vi "None.vi"(8 "error in":errorcluster, 11 "ATM Data":T1={"UI Refs"={"Right Buttons"=refnum, "Left Buttons"=refnum, "User Input"=refnum, "ATM Messages"=refnum, "Left Menu"=refnum, "Right Menu"=refnum, "Enter"=refnum}, "Map"={}, "Login Valid?"=FALSE, "Queue Message"=refnum, "State"=enum."None", "User"={"Pin"="", "First Name"="", "Last Name"="", "Balance"=0.0, "Login Valid?"=FALSE}, "Main States"={"Message"="Initialize", "Data"=variant}}) -> (0 "error out":errorcluster, 3 "ATM Data Out":T1={"UI Refs"={"Right Buttons"=refnum, "Left Buttons"=refnum, "User Input"=refnum, "ATM Messages"=refnum, "Left Menu"=refnum, "Right Menu"=refnum, "Enter"=refnum}, "Map"={}, "Login Valid?"=FALSE, "Queue Message"=refnum, "State"=enum."None", "User"={"Pin"="", "First Name"="", "Last Name"="", "Balance"=0.0, "Login Valid?"=FALSE}, "Main States"={"Message"="Initialize", "Data"=variant}})   [LabVIEW 2020, in "ATM Machine.lvlib"]
uses:
  Cluster - ATM Machine Data.ctl
  Users/khemr/OneDrive/Desktop/Labview Training/CLD/New ATM_KR/ATM Machine/Cluster - Message Cluster.ctl
  Enum - ATM States.ctl
  ATM Machine.lvlib
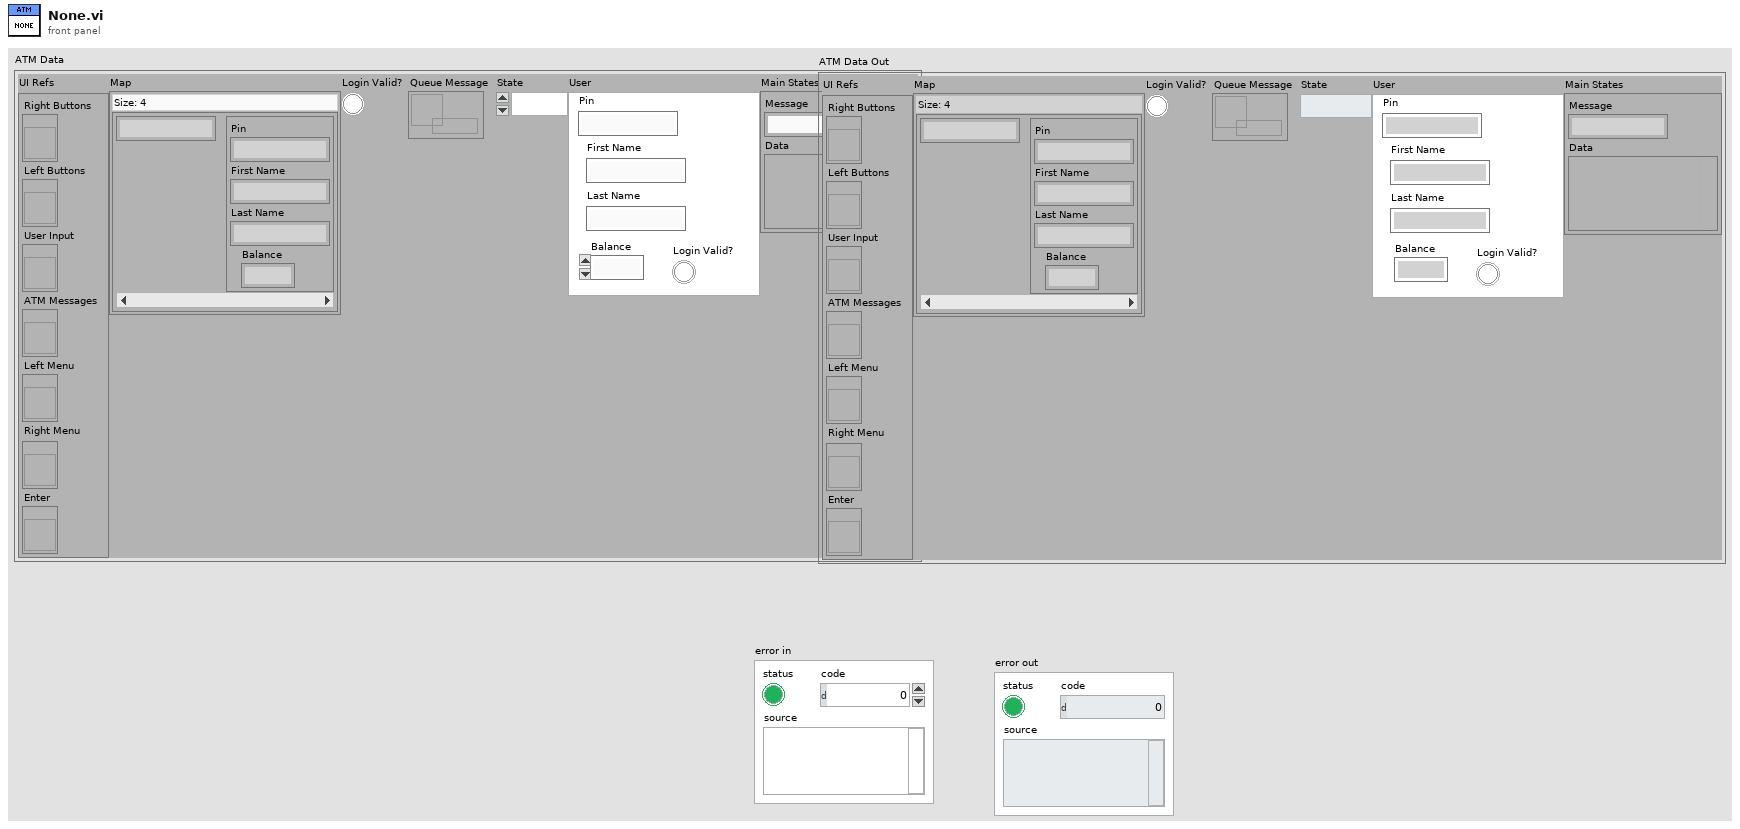
[diagram p1: front panel]
types:
  T1 = typedef "ATM Machine.lvlib/Cluster - ATM Machine Data.ctl" = cluster{"UI Refs":cluster{"Right Buttons":refnum<vi>, "Left Buttons":refnum<vi>, "User Input":refnum<vi>, "ATM Messages":refnum<vi>, "Left Menu":refnum<vi>, "Right Menu":refnum<vi>, "Enter":refnum<vi>}, "Map":map{string, cluster{"Pin":string, "First Name":string, "Last Name":string, "Balance":dbl}}, "Login Valid?":bool, "Queue Message":refnum<queue>, "State":T2, "User":cluster{"Pin":string, "First Name":string, "Last Name":string, "Balance":dbl, "Login Valid?":bool}, "Main States":cluster{"Message":string, "Data":variant}}
  T2 = typedef "ATM Machine.lvlib/Enum - ATM States.ctl" = enum16{"None", "Deposit", "Withdraw", "Card Inserted", "Balance Inquiry", "Return Card and Terminate", "Fast Cash"}
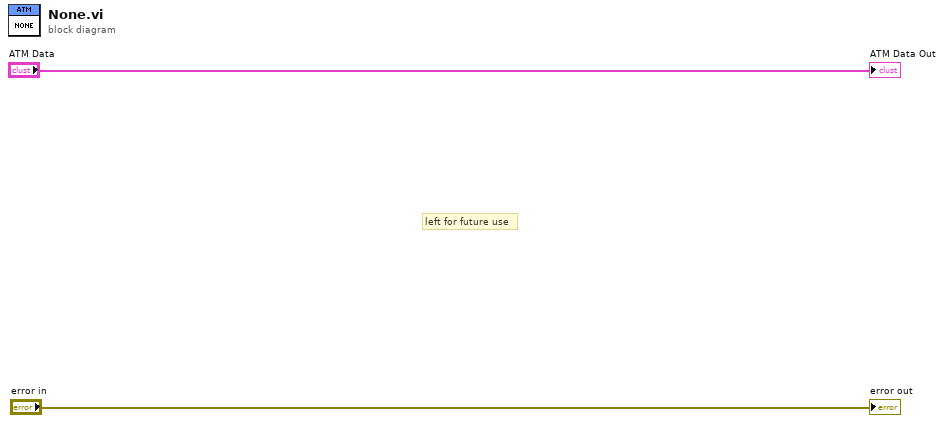
[diagram p0: block diagram]
diagram:
  # "left for future use"
  "ATM Data Out" <- "ATM Data"
  "error out" <- "error in"
